vi "Create Statement from CSV.vi"(8 "error in (no error)":errorcluster, 11 "CSV Entries":string[](array[string])) -> (0 "error out":errorcluster, 3 "Banking Statement.lvclass":refnum<class "Banking Statement.lvclass">)   [LabVIEW 2018, in "Banking Statement.lvclass"]
uses:
  Banking Statement.lvclass
  C:/GitRepos/Filthy-Lucre-Budgetizer/source/support/classes/Statement/Statement.lvclass
  Banking Record/Banking Transaction.lvclass
  C:/GitRepos/Filthy-Lucre-Budgetizer/source/support/classes/Transaction/Transaction.lvclass
  Statement/Statement.lvclass
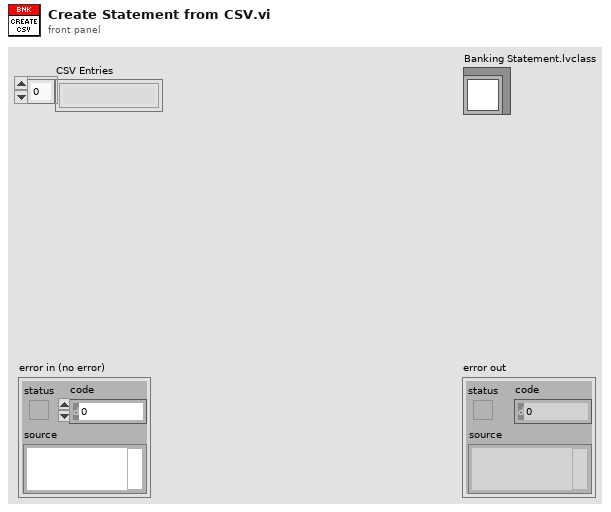
[diagram p1: front panel]
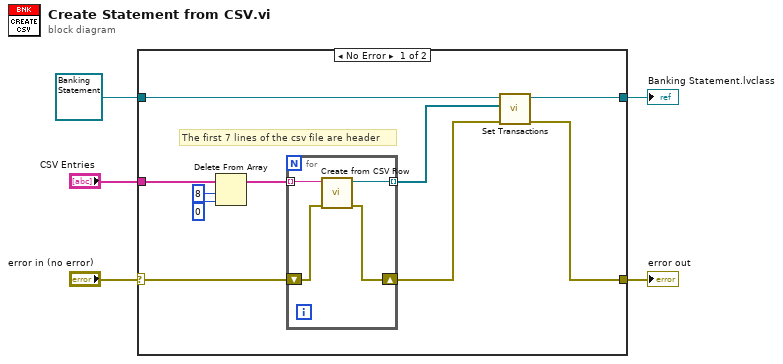
[diagram p0: block diagram]
diagram:
  n1 = case shown="No Error" "error in (no error)" {
    selector: "error in (no error)" -> [w15 w21]
    tunnel: [w6 w21] -> w4
    tunnel: [w9 w20] -> w3
    tunnel: "CSV Entries" -> [w12 _]
    tunnel: refnum<class "Banking Statement.lvclass"> refnum ("Banking Statement.lvclass") -> [w10 w20]
    frame No Error {
      # "The first 7 lines of the csv file are header"
      n2 = Delete From Array(array=w12, length=8, index=0) -> (array with subset deleted=w11:string[])  [unwired: 1 out]
      n3 = for {
        tunnel: w11 -> [w18] mode=indexing
        tunnel: [w19] -> w8 mode=indexing
        shift-right: [w16] -> w7
        shift-left: w15 -> [w17]
        n4 = call "Create from CSV Row.vi"("error in (no error)"=w17, "CSV Row"=w18) -> ("error out"=w16:errorcluster, "Banking Record"=w19:refnum<class "Banking Transaction.lvclass">)  [unwired: 8 in]
      }
      n5 = call "Set Transactions.vi"("error in (no error)"=w7, "Transactions"=w8, "Statement in"=w10) -> ("error out"=w6:errorcluster, "Statement out"=w9:refnum<class "Banking Statement.lvclass">)  [unwired: 7 in]
    }
    frame Error {
    }
  }
  "error out" <- w4
  "Banking Statement.lvclass" <- w3
